vi "FeedbackDecode_20200902.vi"() -> ()   [LabVIEW 2016] (continued)
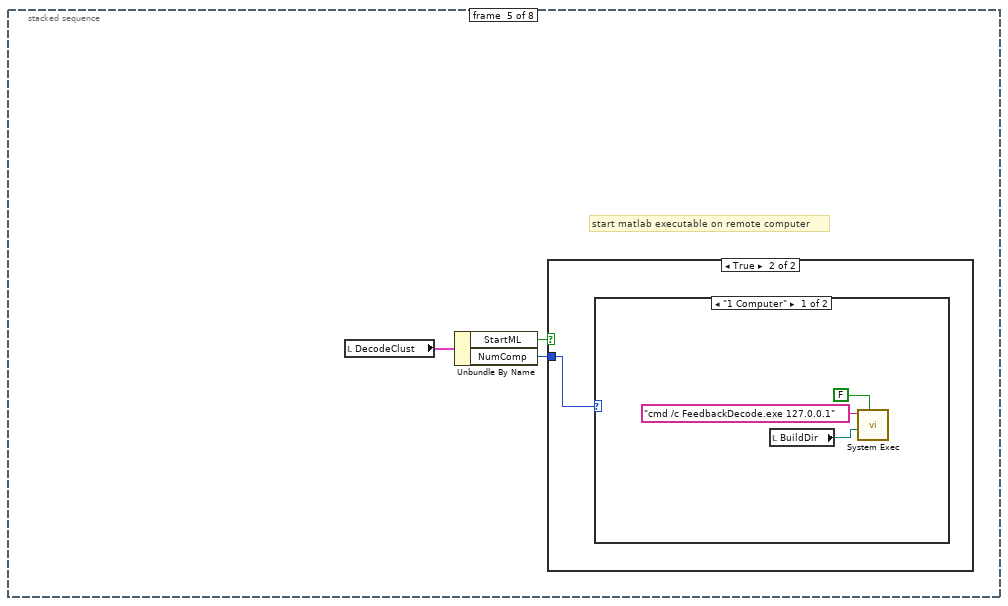
[diagram p17: hidden frame]
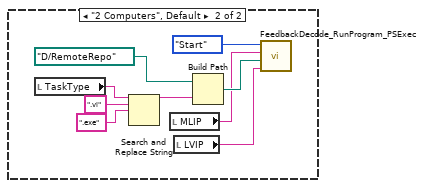
[diagram p19: hidden frame]
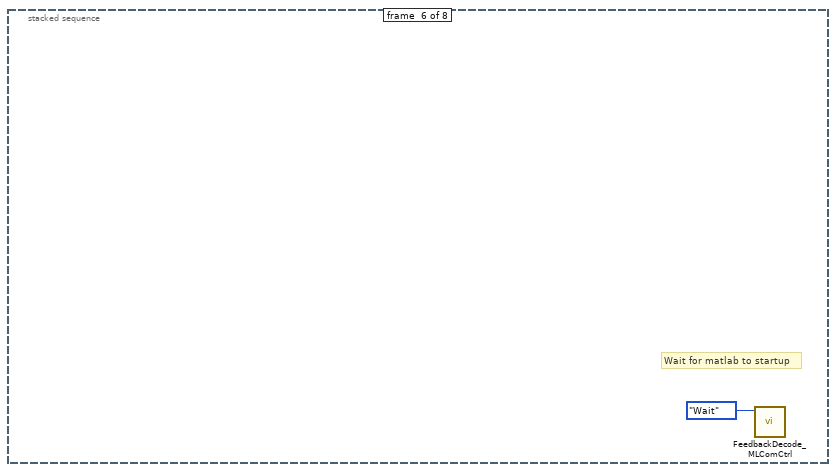
[diagram p20: hidden frame]
